vi "PCIe_6376_Data_Acquisition_Cui.vi"() -> ()   [LabVIEW 2018]
uses:
  <vilib>/DAQmx/read.llb/DAQmx Read (Analog 2D DBL NChan NSamp).vi
  <vilib>/DAQmx/create/channels.llb/DAQmx Create Channel (AI-Voltage-Basic).vi
  <vilib>/DAQmx/configure/timing.llb/DAQmx Timing (Sample Clock).vi
  <vilib>/DAQmx/configure/trigger.llb/DAQmx Reference Trigger (Digital Edge).vi
  <vilib>/DAQmx/miscellaneous.llb/DAQmx Fill In Error Info.vi
  <vilib>/Utility/file.llb/Write Delimited Spreadsheet (DBL).vi
panel:
  out "error out":errorcluster
  out "数值 7":dbl=-10.0
  in  "Channel 7":dbl=10.0 min=1.0 max=10.0
  out "数值 6":dbl=-10.0
  in  "Channel 6":dbl=10.0 min=1.0 max=10.0
  out "数值 5":dbl=-10.0
  in  "Channel 5":dbl=10.0 min=1.0 max=10.0
  out "数值 4":dbl=-10.0
  in  "Channel 4":dbl=10.0 min=1.0 max=10.0
  out "数值 3":dbl=-10.0
  in  "Channel 3":dbl=10.0 min=1.0 max=10.0
  out "数值 2":dbl=-10.0
  in  "Channel 2":dbl=10.0 min=1.0 max=10.0
  out "数值 1":dbl=-10.0
  in  "Channel 1":dbl=10.0 min=1.0 max=10.0
  out "数值":dbl=-10.0
  in  "Channel 0":dbl=10.0 min=1.0 max=10.0
  out "数据存储路径":path=path "E:/dianya/20180627_174521_1000000Hz.dat" caption="文件名"
  in  "触发前采样数":dbl=2000.0 min=2000.0 format="%#_6p"
  out "波形图":dbl[][](graph)
  in  "触发通道":string="PFI0"
  in  "边沿":i32(ring)=10280 items=["Rising"=10280, "Falling"=10171]
  in  "采样率":dbl=1000000.0 min=100.0 max=3570000.0 format="%#_6p"
  in  "触发后采样数":dbl=2000.0 min=2000.0 format="%#_6p"
  # "最大值"
  # "最小值"
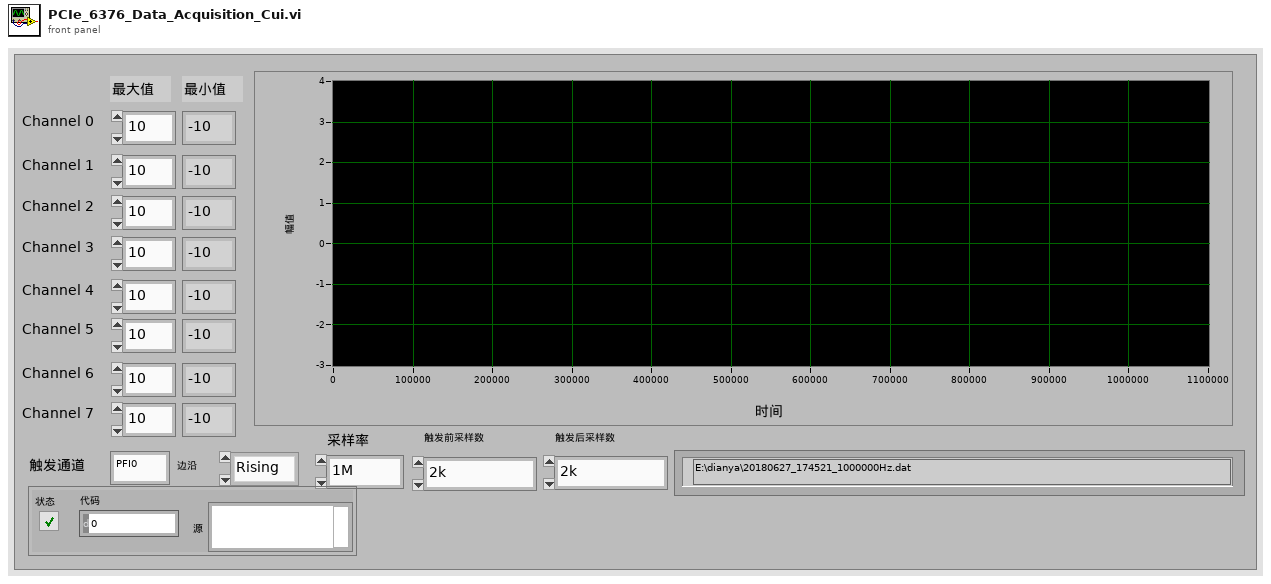
[diagram p1: front panel]
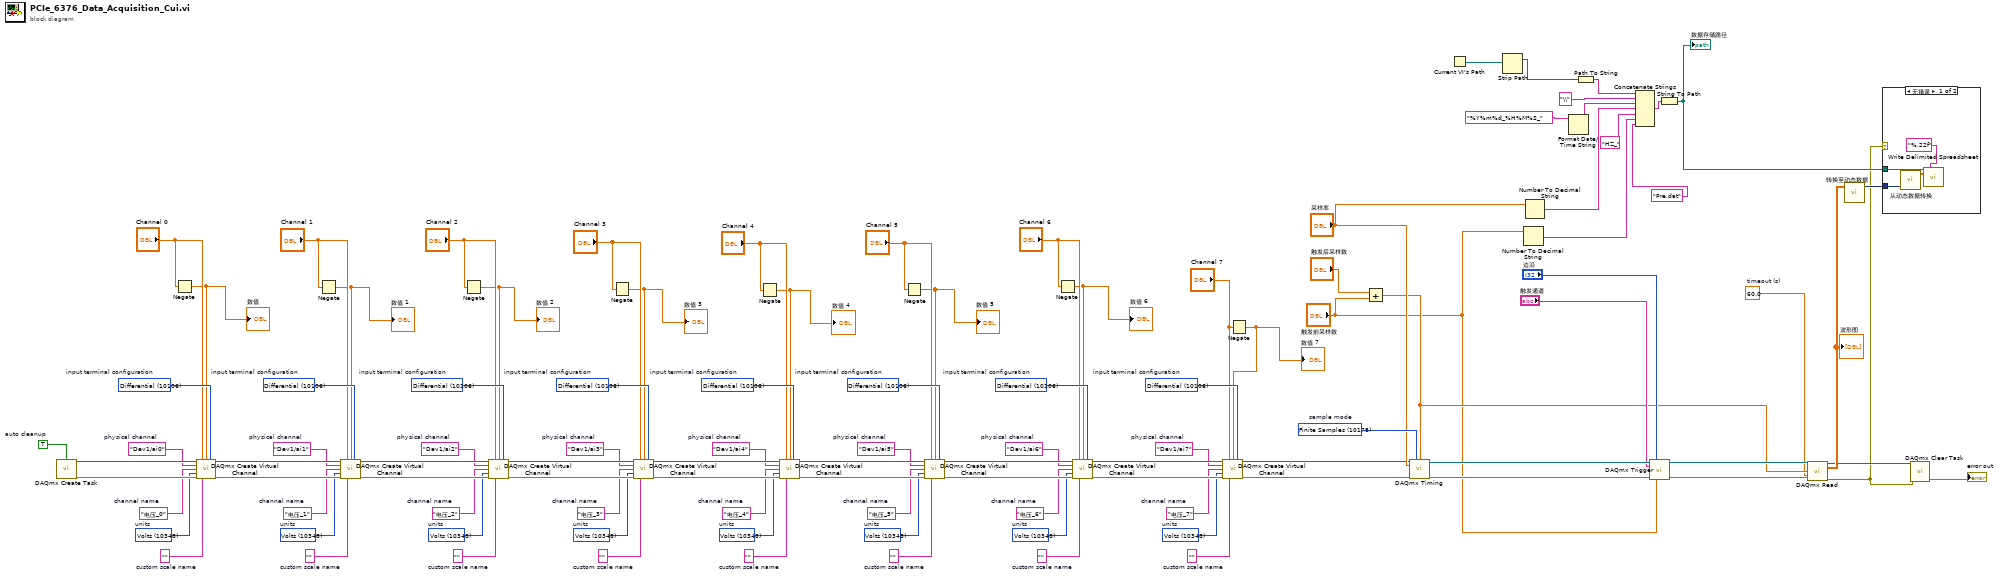
[diagram p0: block diagram]
diagram:
  w28 = 10106 items=["default"=-1, "RSE"=10083, "NRSE"=10078, "Differential"=10106, "Pseudodifferential"=12529]  # input terminal configuration
  w29 = 10348 items=["Volts"=10348, "From Custom Scale"=10065]  # units
  w30 = "电压_7"  # channel name
  w31 = ""  # custom scale name
  w32 = "Dev1/ai7"  # physical channel
  w34 = 10106 items=["default"=-1, "RSE"=10083, "NRSE"=10078, "Differential"=10106, "Pseudodifferential"=12529]  # input terminal configuration
  w35 = 10348 items=["Volts"=10348, "From Custom Scale"=10065]  # units
  w36 = "电压_6"  # channel name
  w38 = ""  # custom scale name
  w39 = "Dev1/ai6"  # physical channel
  w41 = 10106 items=["default"=-1, "RSE"=10083, "NRSE"=10078, "Differential"=10106, "Pseudodifferential"=12529]  # input terminal configuration
  w42 = 10348 items=["Volts"=10348, "From Custom Scale"=10065]  # units
  w43 = "电压_5"  # channel name
  w45 = ""  # custom scale name
  w46 = "Dev1/ai5"  # physical channel
  w48 = 10106 items=["default"=-1, "RSE"=10083, "NRSE"=10078, "Differential"=10106, "Pseudodifferential"=12529]  # input terminal configuration
  w49 = 10348 items=["Volts"=10348, "From Custom Scale"=10065]  # units
  w50 = "电压_4"  # channel name
  w52 = ""  # custom scale name
  w53 = "Dev1/ai4"  # physical channel
  w55 = 10106 items=["default"=-1, "RSE"=10083, "NRSE"=10078, "Differential"=10106, "Pseudodifferential"=12529]  # input terminal configuration
  w56 = 10348 items=["Volts"=10348, "From Custom Scale"=10065]  # units
  w57 = "电压_3"  # channel name
  w59 = ""  # custom scale name
  w60 = "Dev1/ai3"  # physical channel
  w62 = 10106 items=["default"=-1, "RSE"=10083, "NRSE"=10078, "Differential"=10106, "Pseudodifferential"=12529]  # input terminal configuration
  w63 = 10348 items=["Volts"=10348, "From Custom Scale"=10065]  # units
  w64 = "电压_2"  # channel name
  w66 = ""  # custom scale name
  w67 = "Dev1/ai2"  # physical channel
  w69 = 10106 items=["default"=-1, "RSE"=10083, "NRSE"=10078, "Differential"=10106, "Pseudodifferential"=12529]  # input terminal configuration
  w70 = 10348 items=["Volts"=10348, "From Custom Scale"=10065]  # units
  w71 = "电压_1"  # channel name
  w73 = ""  # custom scale name
  w74 = "Dev1/ai1"  # physical channel
  w76 = 10106 items=["default"=-1, "RSE"=10083, "NRSE"=10078, "Differential"=10106, "Pseudodifferential"=12529]  # input terminal configuration
  w77 = 10348 items=["Volts"=10348, "From Custom Scale"=10065]  # units
  w78 = "电压_0"  # channel name
  w80 = ""  # custom scale name
  w81 = "Dev1/ai0"  # physical channel
  w83 = TRUE  # auto cleanup
  w87 = 60.0  # timeout (s)
  w104 = 10178 items=["Finite Samples"=10178, "Continuous Samples"=10123, "Hardware Timed Single Point"=12522]  # sample mode
  n1 = call <vilib>:"DAQmx Create Task.vi"("auto cleanup"=w83) -> ("task out"=w82:refnum<k21>, "error out"=w84:errorcluster)  [unwired: 13 in]
  n2 = Negate(x="Channel 0") -> (-x=w10:dbl)
  "数值" <- w10
  n3 = call-poly <vilib>:"DAQmx Create Virtual Channel.vi"("task in"=w82, "maximum value"="Channel 0", "minimum value"=w10, "input terminal configuration"=w76, "physical channels"=w81, "name to assign"=w78, "units"=w77, "error in"=w84, "custom scale name"=w80) -> ("task out"=w75:refnum<k21>, "error out"=w79:errorcluster)  [unwired: 5 in]
  n4 = Negate(x="Channel 1") -> (-x=w12:dbl)
  "数值 1" <- w12
  n5 = call-poly <vilib>:"DAQmx Create Virtual Channel.vi"("task in"=w75, "maximum value"="Channel 1", "minimum value"=w12, "input terminal configuration"=w69, "physical channels"=w74, "name to assign"=w71, "units"=w70, "error in"=w79, "custom scale name"=w73) -> ("task out"=w68:refnum<k21>, "error out"=w72:errorcluster)  [unwired: 5 in]
  n6 = Negate(x="Channel 2") -> (-x=w14:dbl)
  "数值 2" <- w14
  n7 = call-poly <vilib>:"DAQmx Create Virtual Channel.vi"("task in"=w68, "maximum value"="Channel 2", "minimum value"=w14, "input terminal configuration"=w62, "physical channels"=w67, "name to assign"=w64, "units"=w63, "error in"=w72, "custom scale name"=w66) -> ("task out"=w61:refnum<k21>, "error out"=w65:errorcluster)  [unwired: 5 in]
  n8 = Negate(x="Channel 3") -> (-x=w16:dbl)
  "数值 3" <- w16
  n9 = call-poly <vilib>:"DAQmx Create Virtual Channel.vi"("task in"=w61, "maximum value"="Channel 3", "minimum value"=w16, "input terminal configuration"=w55, "physical channels"=w60, "name to assign"=w57, "units"=w56, "error in"=w65, "custom scale name"=w59) -> ("task out"=w54:refnum<k21>, "error out"=w58:errorcluster)  [unwired: 5 in]
  n10 = Negate(x="Channel 4") -> (-x=w18:dbl)
  "数值 4" <- w18
  n11 = call-poly <vilib>:"DAQmx Create Virtual Channel.vi"("task in"=w54, "maximum value"="Channel 4", "minimum value"=w18, "input terminal configuration"=w48, "physical channels"=w53, "name to assign"=w50, "units"=w49, "error in"=w58, "custom scale name"=w52) -> ("task out"=w47:refnum<k21>, "error out"=w51:errorcluster)  [unwired: 5 in]
  n12 = Negate(x="Channel 5") -> (-x=w20:dbl)
  "数值 5" <- w20
  n13 = call-poly <vilib>:"DAQmx Create Virtual Channel.vi"("task in"=w47, "maximum value"="Channel 5", "minimum value"=w20, "input terminal configuration"=w41, "physical channels"=w46, "name to assign"=w43, "units"=w42, "error in"=w51, "custom scale name"=w45) -> ("task out"=w40:refnum<k21>, "error out"=w44:errorcluster)  [unwired: 5 in]
  n14 = Negate(x="Channel 6") -> (-x=w22:dbl)
  "数值 6" <- w22
  n15 = call-poly <vilib>:"DAQmx Create Virtual Channel.vi"("task in"=w40, "maximum value"="Channel 6", "minimum value"=w22, "input terminal configuration"=w34, "physical channels"=w39, "name to assign"=w36, "units"=w35, "error in"=w44, "custom scale name"=w38) -> ("task out"=w33:refnum<k21>, "error out"=w37:errorcluster)  [unwired: 5 in]
  n16 = Negate(x="Channel 7") -> (-x=w24:dbl)
  "数值 7" <- w24
  n17 = call-poly <vilib>:"DAQmx Create Virtual Channel.vi"("task in"=w33, "maximum value"="Channel 7", "minimum value"=w24, "input terminal configuration"=w28, "physical channels"=w32, "name to assign"=w30, "units"=w29, "error in"=w37, "custom scale name"=w31) -> ("task out"=w27:refnum<k21>, "error out"=w26:errorcluster)  [unwired: 5 in]
  n18 = Add(x="触发后采样数", y="触发前采样数") -> (x+y=w88:dbl)
  n19 = call-poly <vilib>:"DAQmx Timing.vi"("task/channels in"=w27, "sample mode"=w104, "samples per channel"=w88, "rate"="采样率", "error in"=w26) -> ("task out"=w102:refnum<k21>, "error out"=w103:errorcluster)  [unwired: 9 in]
  n20 = Current VI's Path() -> (path=w8:path)
  n21 = Strip Path(path=w8) -> (stripped path=w9:path)  [unwired: 1 out]
  n22 = Number To Decimal String(number="触发前采样数") -> (decimal integer string=w5:string)  [unwired: 1 in]
  n23 = Number To Decimal String(number="采样率") -> (decimal integer string=w92:string)  [unwired: 1 in]
  n24 = Format Date/Time String(time format string (%c)="%Y%m%d_%H%M%S_" ("时间格式字符串(%c)")) -> (date/time string=w96:string)  [unwired: 2 in]
  n25 = Path To String(path=w9) -> (string=w95:string)
  n26 = Concatenate Strings(w95, "\\", w96, w92, "HZ_", w5, "Pre.dat" ("字符串")) -> (w94:string)
  n27 = call-poly <vilib>:"DAQmx Trigger.vi"("task/channels in"=w102, "source"="触发通道", "edge"="边沿", "error in"=w103, "pretrigger samples per channel"="触发前采样数") -> ("task out"=w90:refnum<k21>, "error out"=w89:errorcluster)  [unwired: 9 in]
  n28 = String To Path(string=w94) -> (path=w93:path)
  "数据存储路径" <- w93
  n29 = call-poly <vilib>:"DAQmx Read.vi"("task/channels in"=w90, "number of samples per channel"=w88, "timeout"=w87, "error in"=w89) -> ("task out"=w3:refnum<k21>, "data"=w86:dbl[][], "error out"=w1:errorcluster)  [unwired: 9 in]
  "波形图" <- w86
  n30 = call "转换至动态数据"("2D Array"=w86) -> ("Dynamic Data Type"=w85:dynamicdata)  [unwired: 3 in]
  n31 = case shown="无错误" w1 {
    tunnel: w93 -> [w108 _]
    tunnel: w85 -> [w106 _]
    frame No Error {
      n32 = call "从动态数据转换"("Dynamic Data Type"=w106) -> ("Array"=w105:dbl[][])  [unwired: 3 in]
      n33 = call-poly <vilib>:"Write Delimited Spreadsheet.vi"("file path (dialog if empty)"=w108, "format (%.3f)"="%.22f", "2D data"=w105) -> ()  [unwired: 11 in, 2 out]
    }
    frame Error {
    }
  }
  n34 = call <vilib>:"DAQmx Clear Task.vi"("task in"=w3, "error in"=w1) -> ("error out"=→"error out":errorcluster)  [unwired: 13 in]
